vi "generate_id.vi"(7 "queues":variant, 8 "error in (no error)":errorcluster) -> (0 "error out":errorcluster, 3 "id":string)   [LabVIEW 2015, in "lv-waitgroup.lvlib"]
uses:
  lv-waitgroup.lvlib
  public/_controls/data_error.ctl
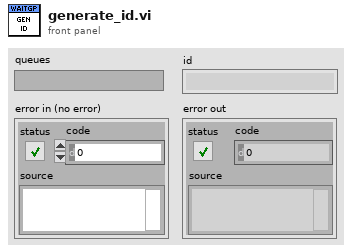
[diagram p1: front panel]
types:
  T1 = typedef "lv-waitgroup.lvlib/data_error.ctl" = enum16{"<data_error>", "unable_to_generate_id", "<null>"}
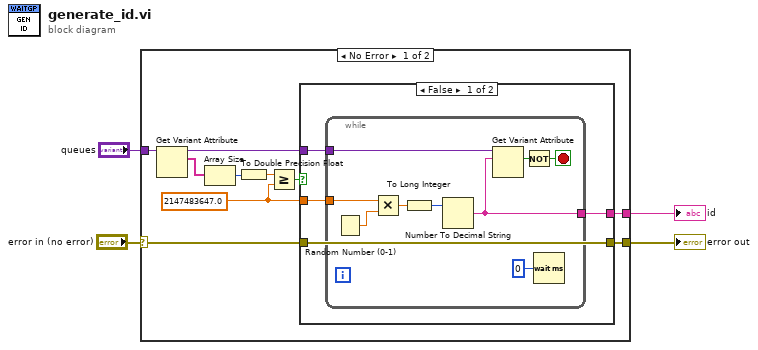
[diagram p0: block diagram]
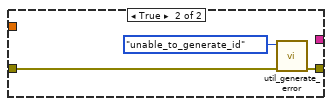
[diagram p2: hidden frame]
diagram:
  n1 = case shown="No Error" "error in (no error)" {
    selector: "error in (no error)" -> [w7 w31]
    tunnel: "queues" -> [w14 _]
    tunnel: [w9 _] -> w3
    tunnel: [w6 w31] -> w1
    frame No Error {
      w10 = 2147483647.0 ("id")
      n2 = Get Variant Attribute(Variant=w14) -> (duplicate Variant=w12:variant, names=w13:string[])  [unwired: 3 in, 2 out]
      n3 = Array Size(array=w13) -> (size(s)=w11:i32)
      n4 = To Double Precision Float(number=w11) -> (double precision float=w5:dbl)
      n5 = Greater Or Equal?(x=w5, y=w10) -> (x >= y?=w8:bool)
      n6 = case shown="False" w8 {
        tunnel: w12 -> [w18 _]
        tunnel: w10 -> [w17 _]
        tunnel: [w16 _] -> w9
        tunnel: w7 -> [w15 w29]
        tunnel: [w15 w28] -> w6
        frame False {
          n7 = while {
            tunnel: w18 -> [w27]
            tunnel: w17 -> [w21]
            tunnel: [w19] -> w16
            stop <- w23 stop-if-true
            n8 = Random Number (0-1)() -> (number: 0 to 1=w26:dbl)
            n9 = Multiply(x=w21, y=w26) -> (x*y=w25:dbl)
            n10 = To Long Integer(number=w25) -> (32bit integer=w20:i32)
            n11 = Number To Decimal String(number=w20) -> (decimal integer string=w19:string)  [unwired: 1 in]
            n12 = Get Variant Attribute(Variant=w27, name=w19) -> (found=w24:bool)  [unwired: 2 in, 3 out]
            n13 = Not(x=w24) -> (.not. x?=w23:bool)
            n14 = Wait (ms)(milliseconds to wait=u32 0) -> ()  [unwired: 1 out]
          }
        }
        frame True {
          n15 = call "util_generate_error.vi"("error in (no error)"=w29, "data_error"=data_error."unable_to_generate_id") -> ("error out"=w28:errorcluster)  [unwired: 9 in]
        }
      }
    }
    frame Error {
    }
  }
  "error out" <- w1
  "id" <- w3
